vi "Read Parameters.vi"(8 "error in (no error)":errorcluster, 11 "Filter in":refnum<class "Filter.lvclass">) -> (0 "error out":errorcluster, 2 "Parameters":T1[](array[typedef]) {"Base Word" format="%04d"; "Address" format="%04x"; "Mask" format="%04x"; "Value" format="%016x"}, 3 "Filter out":refnum<class "Filter.lvclass">)   [LabVIEW 2020, in "BCI-1553 API.lvlib" / "Filter.lvclass"]
uses:
  Filter.lvclass
  Frames & Messages/TypeDefs/Parameter Table Data.ctl
  Frames & Messages/TypeDefs/Scaling Information.ctl
  Filter.lvclass/Filter.ctl
  BCI-1553 API.lvlib
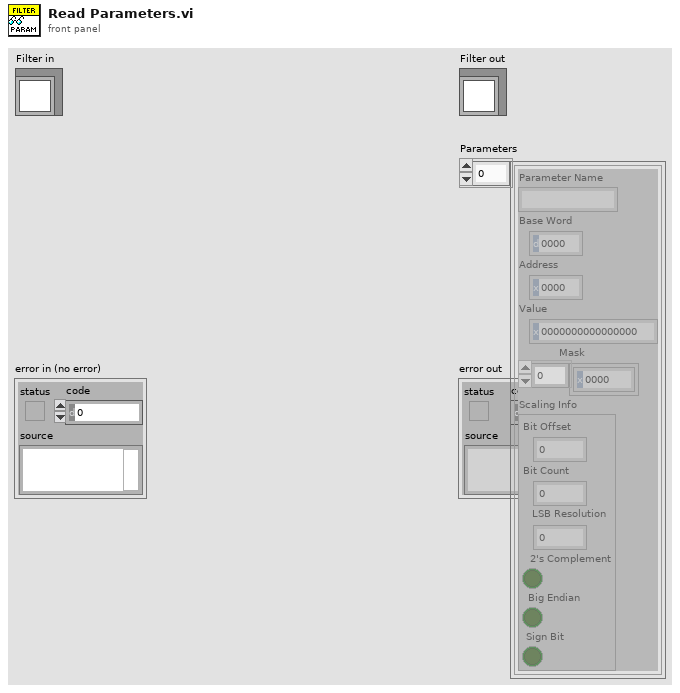
[diagram p1: front panel]
types:
  T1 = typedef "BCI-1553 API.lvlib/Parameter Table Data.ctl" = cluster{"Parameter Name":string, "Base Word":u16, "Address":u16, "Value":u64, "Mask":u16[], "Scaling Info":T2}
  T2 = typedef "BCI-1553 API.lvlib/Scaling Information.ctl" = cluster{"Bit Offset":i32, "Bit Count":i32, "LSB Resolution":dbl, "2's Complement":bool, "Big Endian":bool, "Sign Bit":bool}
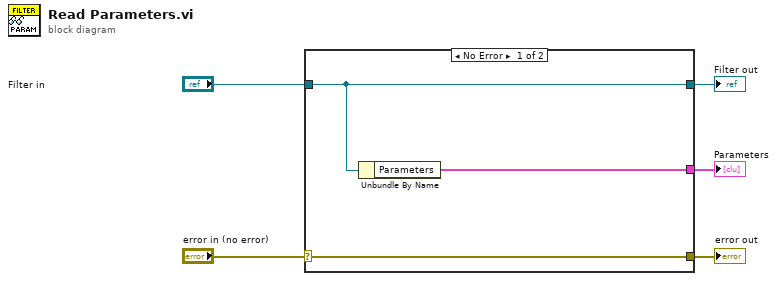
[diagram p0: block diagram]
diagram:
  n1 = case shown="No Error" "error in (no error)" {
    selector: "error in (no error)" -> [w8 w9]
    tunnel: [w8 w9] -> w4
    tunnel: [w7 w10] -> w2
    tunnel: "Filter in" -> [w7 w10]
    tunnel: [w6 _] -> w1
    frame No Error {
      n2 = Unbundle By Name(w7) -> ("Parameters"=w6:T1[])
    }
    frame Error {
    }
  }
  "error out" <- w4
  "Filter out" <- w2
  "Parameters" <- w1
